vi "clustering_xy_sub.vi"(11 "r값 문자열":string) -> (0 "steer":dbl, 1 "전체 관찰용":cluster{cluster{"x":dbl, "y":dbl}[]}[](array[cluster]), 2 "xy 1d clust":cluster{"x":dbl, "y":dbl}[](array[cluster]), 3 "주행 관찰용":cluster{cluster{"x":dbl, "y":dbl}[]}[](array[cluster]))   [LabVIEW 2015]
panel:
  out "XY 그래프 5":cluster{cluster{"x":dbl, "y":dbl}[]}[](graph)
  out "XY 그래프 3":cluster{"x":dbl, "y":dbl}[](graph)
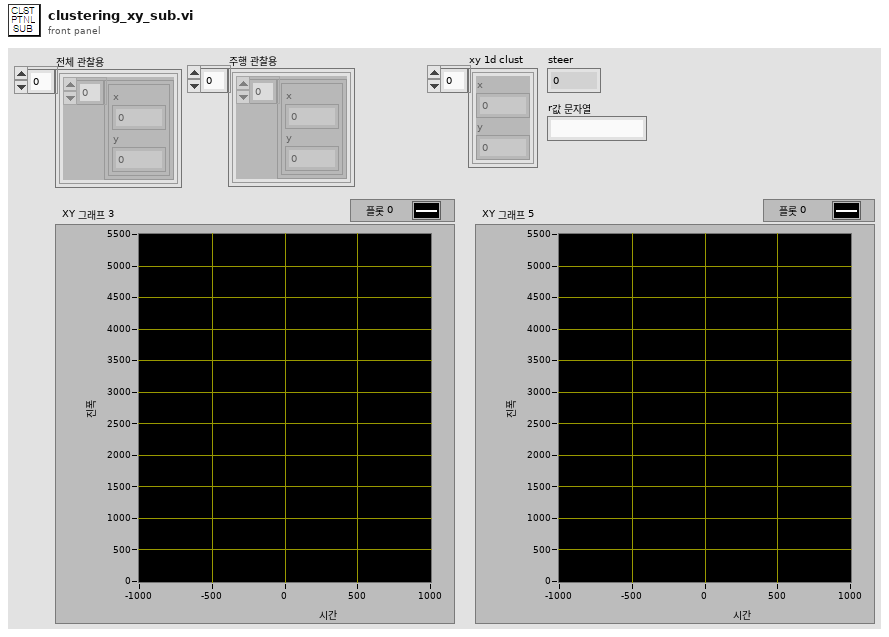
[diagram p1: front panel]
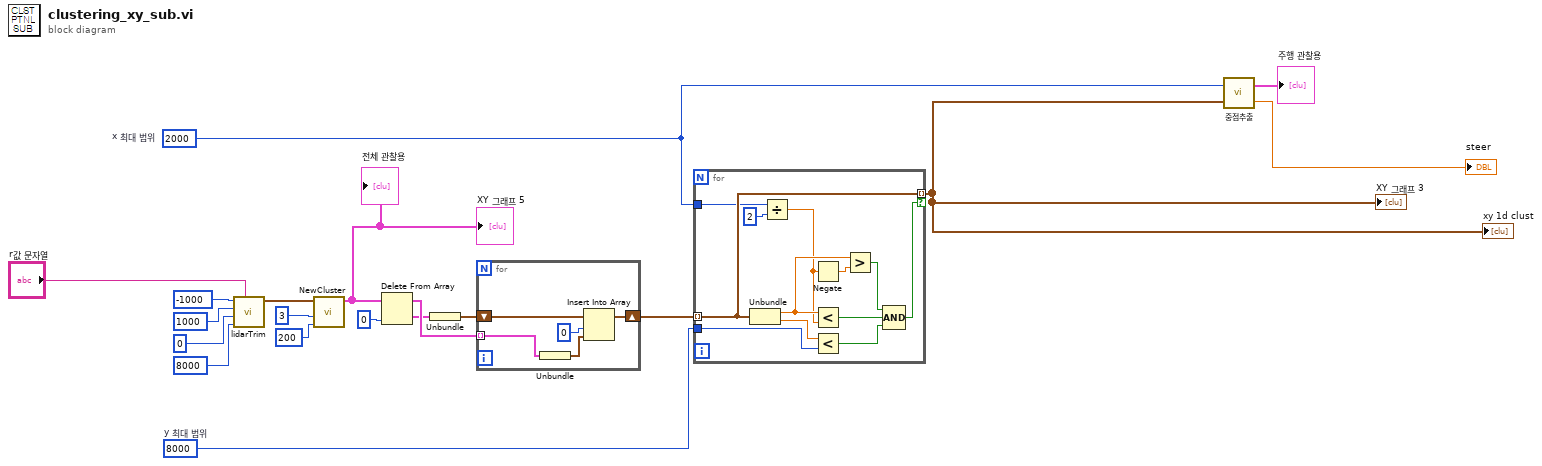
[diagram p0: block diagram]
diagram:
  w12 = 2000  # x 최대 범위
  w14 = 8000  # y 최대 범위
  n1 = call "lidarTrim.vi"("r값 문자열"="r값 문자열", "y+"=8000, "y-"=0, "x+"=1000, "x-"=-1000) -> ("trim된xy"=w9:cluster{"x":dbl, "y":dbl}[])  [unwired: 6 in]
  n2 = call "NewCluster.vi"("R_th"=200, "군집 원소 최수 개수"=3, "x,y 배열"=w9) -> ("클러스터링된 점 배열"=w1:cluster{cluster{"x":dbl, "y":dbl}[]}[])  [unwired: 8 in]
  "XY 그래프 5" <- w1
  "전체 관찰용" <- w1
  n3 = Delete From Array(array=w1, index=0 ("인덱스")) -> (deleted portion=w16:cluster{cluster{"x":dbl, "y":dbl}[]}, array with subset deleted=w19:cluster{cluster{"x":dbl, "y":dbl}[]}[])  [unwired: 1 in]
  n4 = Unbundle(w16) -> (w17:cluster{"x":dbl, "y":dbl}[])
  n5 = for {
    tunnel: w19 -> [w24] mode=indexing
    shift-right: [w21] -> w15
    shift-left: w17 -> [w20]
    n6 = Unbundle(w24) -> (w23:cluster{"x":dbl, "y":dbl}[])
    n7 = Insert Into Array(array=w20, index=0 ("인덱스"), new element=w23) -> (w21:cluster{"x":dbl, "y":dbl}[])
  }
  n8 = for {
    tunnel: w15 -> [w34] mode=indexing
    tunnel: w12 -> [w33]
    tunnel: w14 -> [w35]
    tunnel: [w34] -> w13 mode=indexing if=w25
    n9 = Unbundle(w34) -> ("x"=w31:dbl, "y"=w36:dbl)
    n10 = Divide(x=w33, y=2) -> (x/y=w29:dbl)
    n11 = Negate(x=w29) -> (-x=w30:dbl)
    n12 = Less?(x=w31, y=w29) -> (x < y?=w27:bool)
    n13 = Less?(x=w36, y=w35) -> (x < y?=w28:bool)
    n14 = Greater?(x=w31, y=w30) -> (0:w26:bool)
    n15 = Compound Arithmetic op=AND ("복합 연산")(w26, w27, w28) -> (w25:bool)
  }
  "XY 그래프 3" <- w13
  "xy 1d clust" <- w13
  n16 = call "중점추출.vi"("x,y 배열"=w13, "x범위"=w12) -> ("steer"=→"steer":dbl, "주행 관찰용"=→"주행 관찰용":cluster{cluster{"x":dbl, "y":dbl}[]}[])
